vi "GetTempParam.vi"(8 "error in (no error)":errorcluster, 11 "hcam in":i16) -> (0 "error out":errorcluster, 2 "TSetpointReadback(degC/100)":i16, 3 "hcam out":i16)   [LabVIEW 2013]
uses:
  PARAM_ID_TypDef.ctl
  GetParameterValue(I16).vi
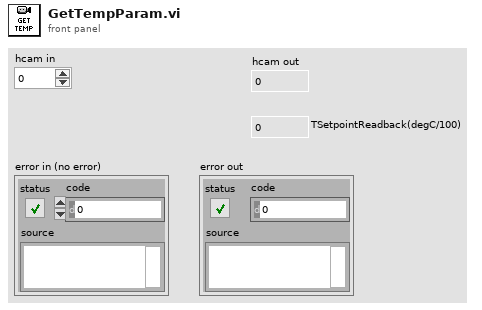
[diagram p1: front panel]
types:
  T1 = typedef "PARAM_ID_TypDef.ctl" = u32
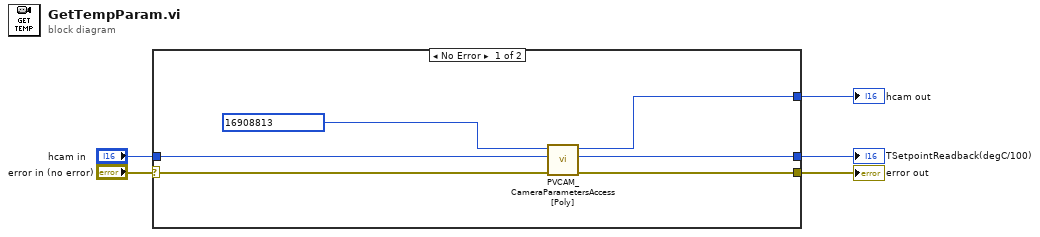
[diagram p0: block diagram]
diagram:
  n1 = case shown="No Error" "error in (no error)" {
    selector: "error in (no error)" -> [w7 w13]
    tunnel: [w11 w13] -> w5
    tunnel: "hcam in" -> [w6 w12]
    tunnel: [w9 _] -> w3
    tunnel: [w8 w12] -> w2
    frame No Error {
      n2 = call-poly "PVCAM_CameraParametersAccess[Poly].vi"("error in (no error)"=w7, "hcam in"=w6, "Param ID (Ring)"=T1 16908813) -> ("error out"=w11:errorcluster, "ParameterValue"=w9:i16, "hcam out"=w8:i16)  [unwired: 6 in]
    }
    frame Error {
    }
  }
  "TSetpointReadback(degC/100)" <- w3
  "error out" <- w5
  "hcam out" <- w2
